vi "display node data.vi"(8 "error in":errorcluster, 11 "NISE_CEF_serializable node in":refnum<class "NISE_CEF_serializable node.lvclass">) -> (0 "error out":errorcluster, 3 "NISE_CEF_serializable node out":refnum<class "NISE_CEF_serializable node.lvclass">)   [LabVIEW 2013, in "NISE_CEF_serializable node.lvclass"]
uses:
  NISE_CEF_serializable node.lvclass
panel:
  in  "OK":bool
  out "node info":string
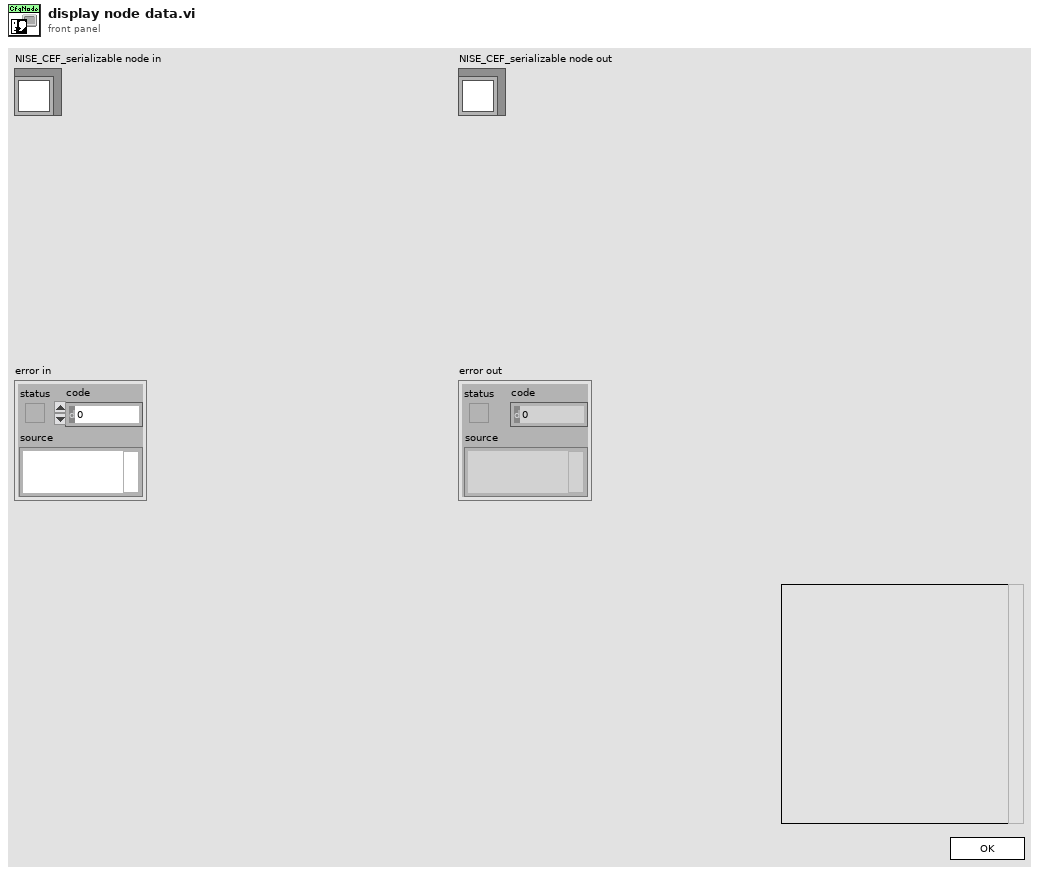
[diagram p1: front panel]
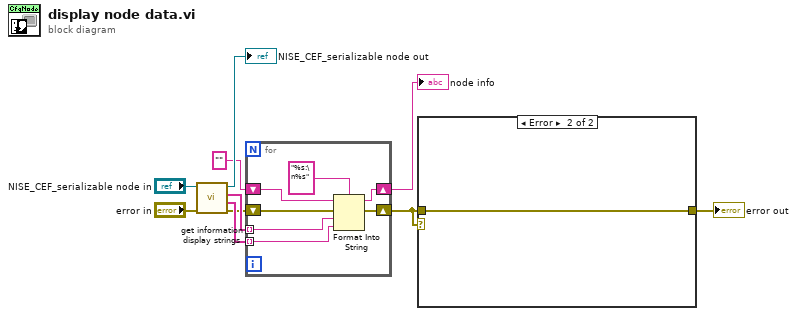
[diagram p0: block diagram]
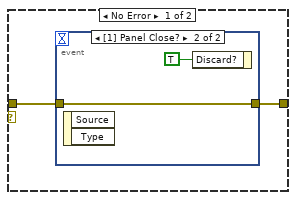
[diagram p2: hidden frame]
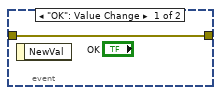
[diagram p3: hidden frame]
diagram:
  n1 = call-dynamic "get information display strings.vi"("error in"="error in", "NISE_CEF_serializable node in"="NISE_CEF_serializable node in") -> ("error out"=w4:errorcluster, "Data"=w6:string[], "Labels"=w7:string[], "NISE_CEF_serializable node out"=→"NISE_CEF_serializable node out":refnum<class "NISE_CEF_serializable node.lvclass">)  [unwired: 6 in]
  n2 = for {
    tunnel: w7 -> [w17] mode=indexing
    tunnel: w6 -> [w16] mode=indexing
    shift-right: [w14] -> w3
    shift-left: "" -> [w13]
    shift-right: [w12] -> w1
    shift-left: w4 -> [w11]
    n3 = Format Into String(format string="%s:\n%s", initial string=w13, error in=w11, w17, w16) -> (resulting string=w14:string, error out=w12:errorcluster)
  }
  "node info" <- w3
  n4 = case shown="Error" w1 {
    tunnel: [w19 w23] -> w2
    tunnel: w1 -> [w18 w23]
    frame No Error {
      n5 = event shown="[1] Panel Close?" {
        selector: _ -> [_ _]
        dyn-events: _ -> [_ _]
        timeout: _ -> [_ _]
        tunnel: [w20 w21] -> w19
        tunnel: w18 -> [w20 w21]
        event "OK": Value Change {
          n6 = event-data() -> ()  [unwired: 1 in, 1 out]
        }
        event Panel Close? {
          n7 = event-data() -> ()  [unwired: 1 in, 2 out]
          n8 = event-data("Discard?"=TRUE) -> ()  [unwired: 1 in, 1 out]
        }
      }
    }
    frame Error {
    }
  }
  "error out" <- w2
